vi "Read Client type.vi"(8 "error in (no error)":errorcluster, 11 "RP Instrument in":refnum<class "RP Instrument.lvclass">) -> (0 "error out":errorcluster, 2 "Client type":enum16{"Control", "Reciever", "Transmitter"}(ring), 3 "RP Instrument out":refnum<class "RP Instrument.lvclass">)   [LabVIEW 2015, in "RP Instrument.lvclass"]
uses:
  RP Instrument.lvclass
  RP Instrument.lvclass/RP Instrument.ctl
  RP Communicator/RP Communicator.lvclass/RP Communicator.ctl
  RP Communicator/RP Communicator.lvclass
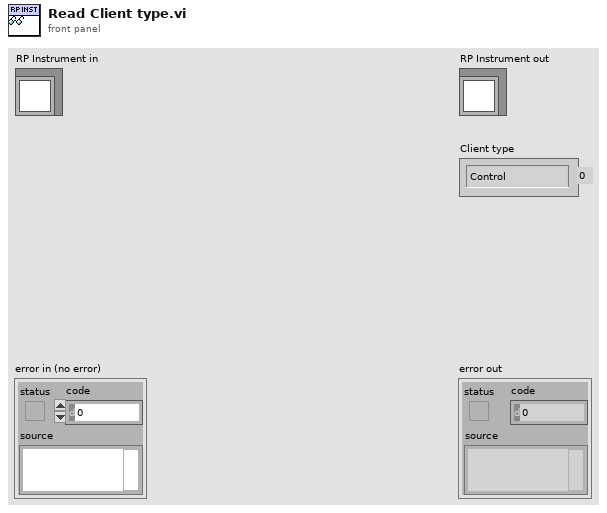
[diagram p1: front panel]
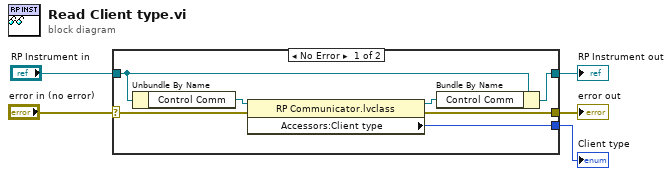
[diagram p0: block diagram]
diagram:
  n1 = case shown="No Error" "error in (no error)" {
    selector: "error in (no error)" -> [w9 w13]
    tunnel: [w8 w13] -> w4
    tunnel: [w7 w14] -> w2
    tunnel: "RP Instrument in" -> [w12 w14]
    tunnel: [w10 _] -> w1
    frame No Error {
      n2 = Unbundle By Name(w12) -> ("Control Comm"=w11:refnum<class "RP Communicator.lvclass">)
      n3 = property class="RP Communicator.lvclass"(reference=w11, error in=w9) -> (reference out=w6:refnum<class "RP Communicator.lvclass">, error out=w8:errorcluster, "Accessors:Client type"=w10:enum16{"Control", "Reciever", "Transmitter"})
      n4 = Bundle By Name(cluster=w12, "Control Comm"=w6) -> (w7:refnum<class "RP Instrument.lvclass">)
    }
    frame Error {
    }
  }
  "error out" <- w4
  "RP Instrument out" <- w2
  "Client type" <- w1
